vi "DAQ.vi"() -> ()   [LabVIEW 2024]
uses:
  <vilib>/Instr/_visa.llb/VISA Configure Serial Port (Instr).vi
panel:
  in  "Tab Control":enum32{"Page 1", "Page 2"}(tab)
  out "BT":dbl(knob) scale=0.0..4096.0
  in  "stop":bool
  in  "VISA resource name":refnum<visa-resource-name>
  out "Temperature":dbl(slide) scale=0.0..100.0
  out "Humidity":dbl(slide) scale=0.0..100.0
  out "Temp":dbl
  out "Hum":dbl
  out "BT":dbl
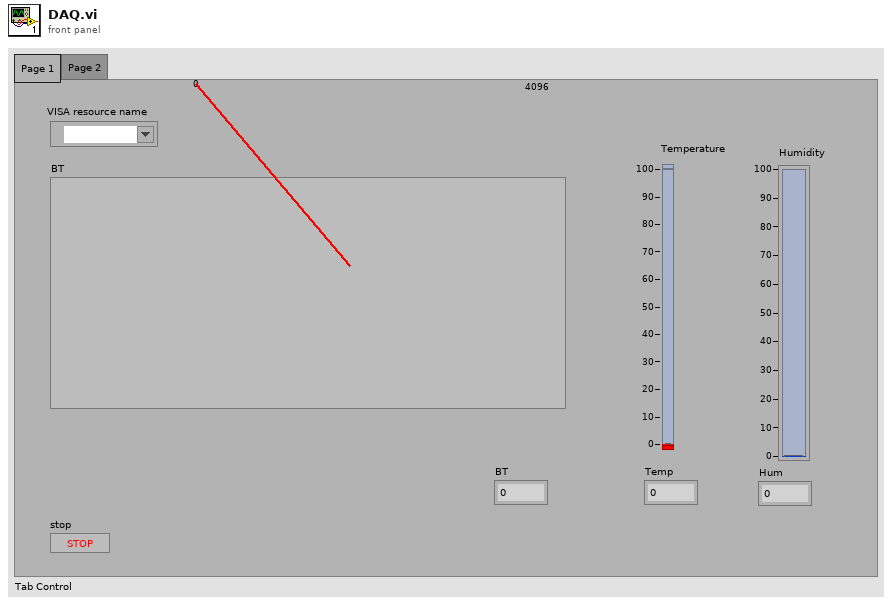
[diagram p1: front panel]
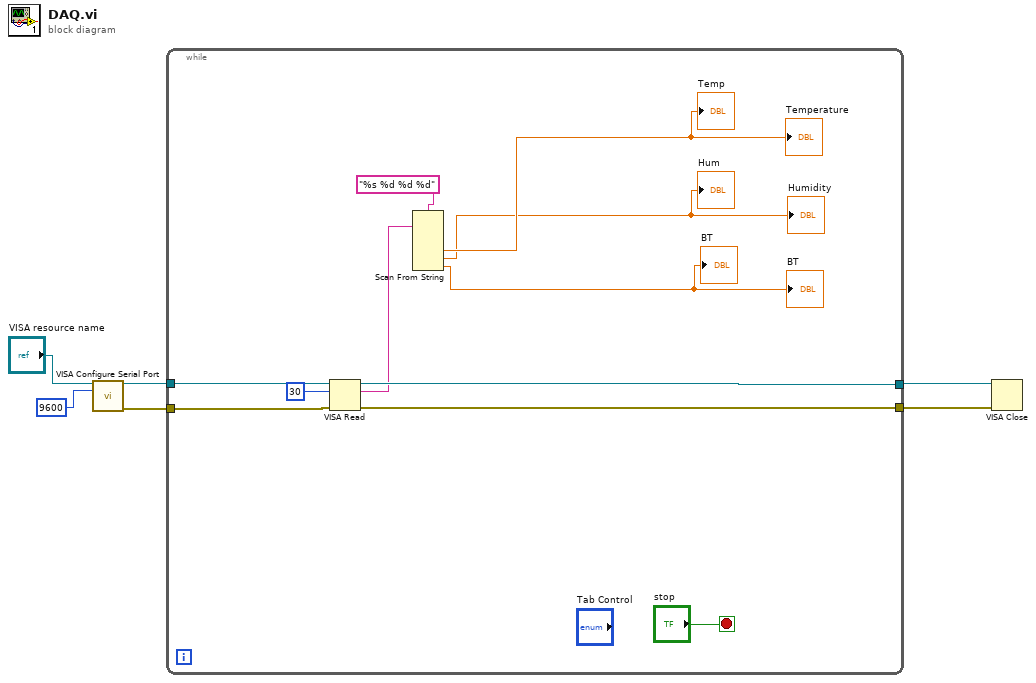
[diagram p0: block diagram]
diagram:
  n1 = call-poly "VISA Configure Serial Port"("VISA resource name"="VISA resource name", "baud rate (9600)"=u32 9600) -> ("VISA resource name out"=w5:refnum<visa-resource-name>, "error out"=w4:errorcluster)  [unwired: 12 in]
  n2 = while {
    tunnel: w5 -> [w16]
    tunnel: w4 -> [w15]
    tunnel: [w13] -> w3
    tunnel: [w12] -> w2
    stop <- "stop" stop-if-true
    n3 = VISA Read(VISA resource name=w16, byte count=u32 30, error in (no error)=w15) -> (VISA resource name out=w13:refnum<visa-resource-name>, read buffer=w10:string, error out=w12:errorcluster)  [unwired: 1 out]
    n4 = Scan From String(format string="%s %d %d %d", input string=w10) -> (output 2=→"Temperature" →"Temp":dbl, output 3=→"Humidity" →"Hum":dbl, output 4=→"BT" →"BT":dbl)  [unwired: 7 in, 3 out]
  }
  n5 = VISA Close(VISA resource name=w3, error in (no error)=w2) -> ()  [unwired: 1 out]
